vi "gwyscan create path regular.vi"(0 "xypos":dbl[](array[numeric]), 1 "yreal":dbl, 2 "yoffset":dbl, 3 "direction":u32(ring) items=["GWYSCAN_DIRECTION_FORWARD", "GWYSCAN_DIRECTION_REVERSE", "GWYSCAN_DIRECTION_BOTH", "GWYSCAN_DIRECTION_BIDIRECTIONAL"], 5 "xres":i32, 7 "yres":i32, 9 "xreal":dbl, 11 "error in (no error)":errorcluster, 12 "xoffset":dbl, 13 "angle":dbl) -> (4 "xypos 2":dbl[](array[numeric]), 6 "function return":i32, 15 "error out":errorcluster)   [LabVIEW 2016, in "libgwyscan.lvlib"]
doc: "GWYSCANDLL_API int gwyscan_create_path_regular(double *xypos, int xres, int yres, double xreal, double yreal, double xoffset, double yoffset, double angle, GwyscanDirection direction);"
uses:
  libgwyscan.lvlib
  libgwyscan.dll
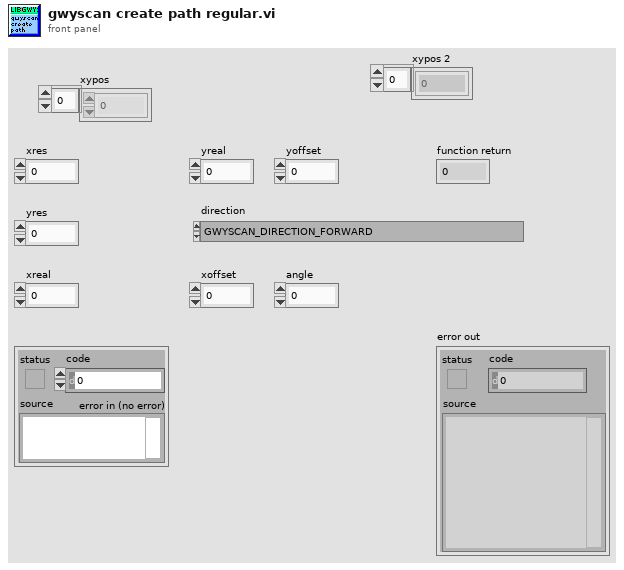
[diagram p1: front panel]
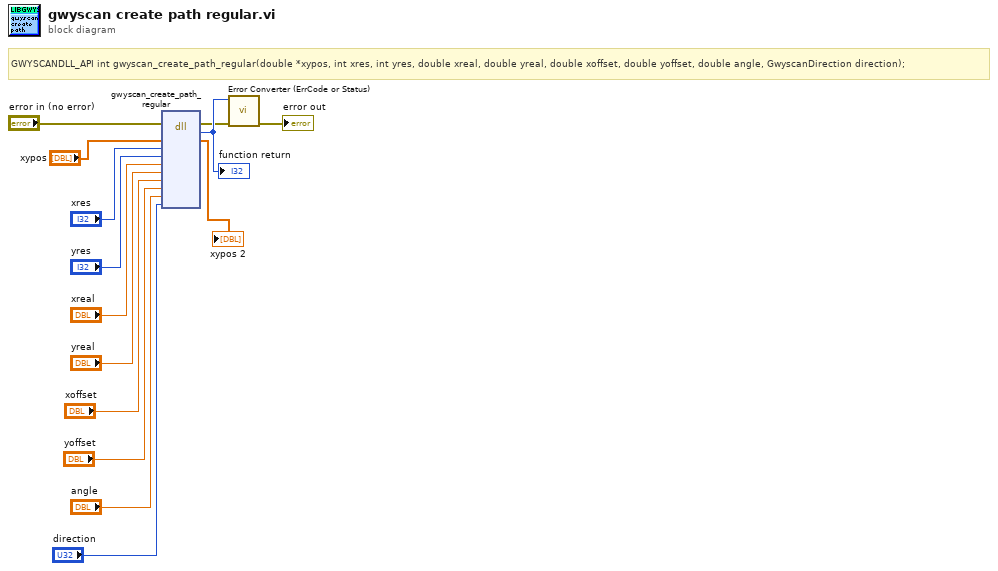
[diagram p0: block diagram]
diagram:
  # "GWYSCANDLL_API int gwyscan_create_path_regular(double *xypos, int xres, int yres, double xreal, double yreal, double xoffset, double yoffset, double angle, GwyscanDirection direction);"
  n1 = dll-call lib="PTH2abs CUsersCharlÃ¨ne BrillardDesktoplbni-lbniAFMController-BetaVersionv2.0.16-20190611 libgwyscan-1.2-labview2015-win32libgwyscan.*" fn="gwyscan_create_path_regular"(error in="error in (no error)", "xypos"="xypos", "xres"="xres", "yres"="yres", "xreal"="xreal", "yreal"="yreal", "xoffset"="xoffset", "yoffset"="yoffset", "angle"="angle", "direction"="direction") -> (error out=w2:errorcluster, "return type"=w14:i32, "xypos"=→"xypos 2":dbl[])  [unwired: 10 in, 1 out]
  "function return" <- w14
  n2 = call "Error Converter (ErrCode or Status).vi"("error in (no error)"=w2, "error code"=w14) -> ("error out"=→"error out":errorcluster)  [unwired: 9 in]
